vi "Modulation Information Set.vi"(8 "error in (no error)":errorcluster, 9 "Modulation Type":u16(ring) items=["Multiplication", "Addition"], 10 "Select Output to Modulate":i8(ring) items=["None", "Voltage", "Current"], 11 "VISA session":refnum<visa-resource-name>) -> (0 "error out":errorcluster, 3 "dup VISA session":refnum<visa-resource-name>)   [LabVIEW 2011, in "Magna PSU.lvlib"]
uses:
  Magna PSU.lvlib
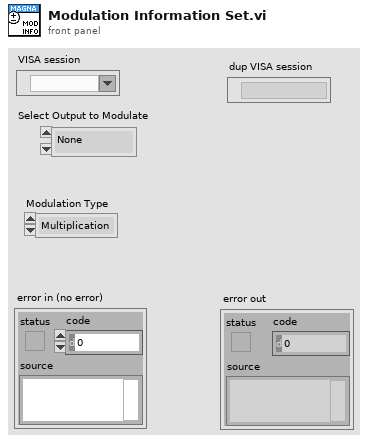
[diagram p1: front panel]
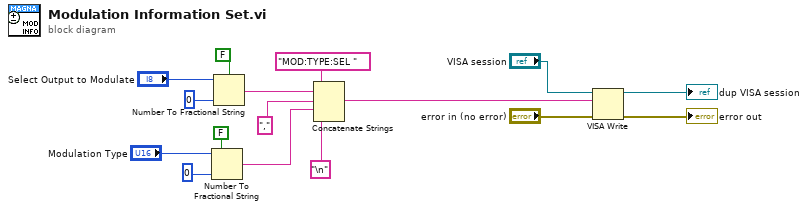
[diagram p0: block diagram]
diagram:
  n1 = Number To Fractional String(use system decimal point (T)=FALSE, number="Modulation Type", precision (6)=0) -> (F-format string=w3:string)  [unwired: 1 in]
  n2 = Number To Fractional String(use system decimal point (T)=FALSE, number="Select Output to Modulate", precision (6)=0) -> (F-format string=w5:string)  [unwired: 1 in]
  n3 = Concatenate Strings("MOD:TYPE:SEL ", w5, ",", w3, "\n") -> (w11:string)
  n4 = VISA Write(VISA resource name="VISA session", write buffer=w11, error in (no error)="error in (no error)") -> (VISA resource name out=→"dup VISA session":refnum<visa-resource-name>, error out=→"error out":errorcluster)  [unwired: 1 out]
